vi "franch_LLSE.vi"(4 "error in (no error)":errorcluster, 5 "b":cdb[](array[numeric]), 7 "A":cdb[][](array[numeric]) format="%0.2f") -> (0 "error out":errorcluster, 2 "mean square error":dbl, 3 "x.estimate":cdb[](array[numeric]))   [LabVIEW 2012]
uses:
  <vilib>/Analysis/baseanly.llb/Complex A x B.vi
  <vilib>/Analysis/baseanly.llb/Complex Inverse Matrix.vi
  <vilib>/Analysis/baseanly.llb/Complex A x Vector.vi
  <vilib>/Analysis/_algsub.llb/Complex Vector Norm.vi
  <vilib>/Analysis/NI_AALBase.lvlib
  <vilib>/Analysis/NI_AALPro.lvlib
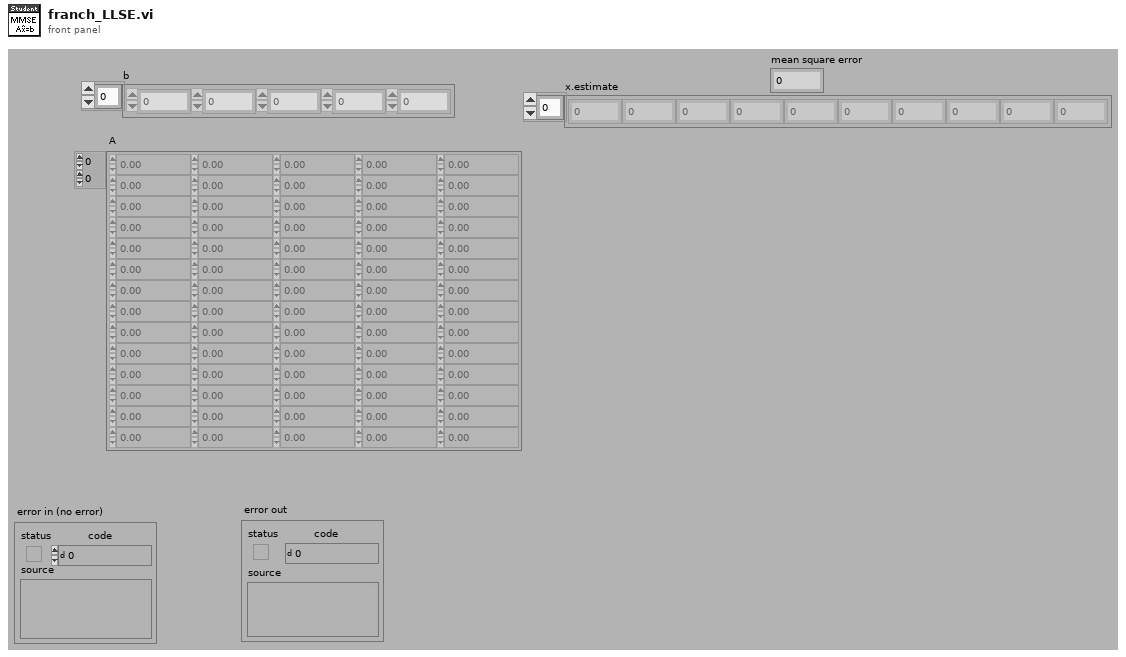
[diagram p1: front panel]
types:
  T1 = typedef "NI_Matrix.lvlib/ComplexMatrix.ctl" = cdb[][]
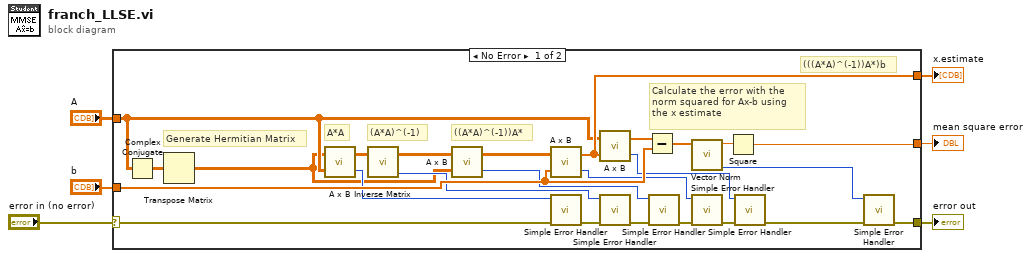
[diagram p0: block diagram]
diagram:
  n1 = case shown="No Error" "error in (no error)" {
    selector: "error in (no error)" -> [w21 w32]
    tunnel: [w28 _] -> w6
    tunnel: [w22 _] -> w2
    tunnel: "A" -> [w25 _]
    tunnel: "b" -> [w24 _]
    tunnel: [w9 w32] -> w1
    frame No Error {
      # "Calculate the error with the\nnorm squared for Ax-b using\nthe x estimate"
      # "(((A*A)^(-1))A*)b"
      # "((A*A)^(-1))A*"
      # "(A*A)^(-1)"
      # "A*A"
      # "Generate Hermitian Matrix"
      n2 = Complex Conjugate(1:w25) -> (0:w8:cdb[][])
      n3 = Transpose Matrix(1:w8) -> (0:w7:cdb[][])
      n4 = call-poly <vilib>:"A x B.vi"("B"=w25, "A"=w7) -> ("error"=w20:i32, "A x B"=w31:T1)
      n5 = call-poly <vilib>:"Inverse Matrix.vi"("Input Matrix"=w31) -> ("error"=w19:i32, "Inverse Matrix"=w30:T1)  [unwired: 1 in]
      n6 = call-poly <vilib>:"A x B.vi"("B"=w7, "A"=w30) -> ("error"=w18:i32, "A x B"=w29:T1)
      n7 = call-poly <vilib>:"A x B.vi"("Vector"=w24, "A"=w29) -> ("error"=w17:i32, "A x Vector"=w28:cdb[])
      n8 = call <vilib>:"Simple Error Handler.vi"("error code (no error:0)"=w20, "error in (no error)"=w21) -> ("error out"=w14:errorcluster)  [unwired: 3 in, 4 out]
      n9 = call-poly <vilib>:"A x B.vi"("Vector"=w28, "A"=w25) -> ("error"=w16:i32, "A x Vector"=w27:cdb[])
      n10 = call <vilib>:"Simple Error Handler.vi"("error code (no error:0)"=w19, "error in (no error)"=w14) -> ("error out"=w13:errorcluster)  [unwired: 3 in, 4 out]
      n11 = Subtract ("Subtract.vi")(x=w27, y=w24) -> (x-y=w26:cdb[])
      n12 = call <vilib>:"Simple Error Handler.vi"("error code (no error:0)"=w18, "error in (no error)"=w13) -> ("error out"=w12:errorcluster)  [unwired: 3 in, 4 out]
      n13 = call-poly <vilib>:"Vector Norm.vi"("Input Vector"=w26) -> ("error"=w15:i32, "norm"=w23:dbl)  [unwired: 9 in]
      n14 = call <vilib>:"Simple Error Handler.vi"("error code (no error:0)"=w17, "error in (no error)"=w12) -> ("error out"=w11:errorcluster)  [unwired: 3 in, 4 out]
      n15 = Square(x=w23) -> (x^2=w22:dbl)
      n16 = call <vilib>:"Simple Error Handler.vi"("error code (no error:0)"=w16, "error in (no error)"=w11) -> ("error out"=w10:errorcluster)  [unwired: 3 in, 4 out]
      n17 = call <vilib>:"Simple Error Handler.vi"("error code (no error:0)"=w15, "error in (no error)"=w10) -> ("error out"=w9:errorcluster)  [unwired: 3 in, 4 out]
    }
    frame Error {
    }
  }
  "mean square error" <- w2
  "x.estimate" <- w6
  "error out" <- w1
